vi "Read GPS Data.vi"(0 "VISA resource name":refnum<visa-resource-name>, 5 "Timeout (3000 ms)":u32=3000, 11 "error in (no error)":errorcluster) -> (2 "Speed Over Ground (knots)":dbl, 3 "Bearing (°)":dbl, 4 "VISA resource name out":refnum<visa-resource-name>, 6 "Time Stamp":timestamp, 8 "Latitude (°)":dbl, 10 "Longitude (°)":dbl, 14 "Altitude (m)":dbl, 15 "error out":errorcluster)   [LabVIEW 2011, in "u-blox 5 Series.lvlib"]
doc: "Reads common GPS information from the u-blox device. This VI reads time, longitude, latitude, altitude, speed, and bearing. See u-blox 5 Series Acquire and Chart GPS Data.vi for an example of how it is used."
uses:
  u-blox 5 Series.lvlib
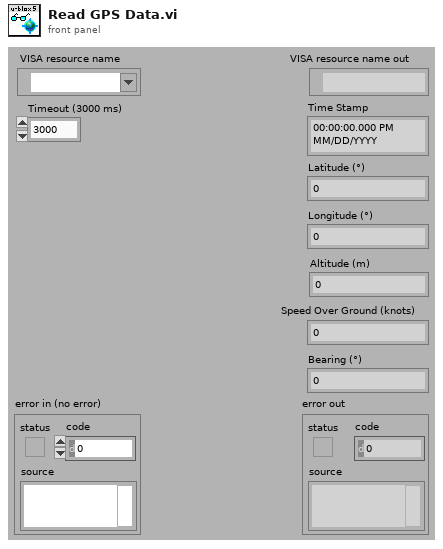
[diagram p1: front panel]
types:
  T1 = cluster{"oldest read timestamp":timestamp, "latitude (deg)":dbl, "longitude (deg)":dbl, "ground speed (knots)":dbl, "true track angle (deg)":dbl, "altitude above mean sea level (m)":dbl}
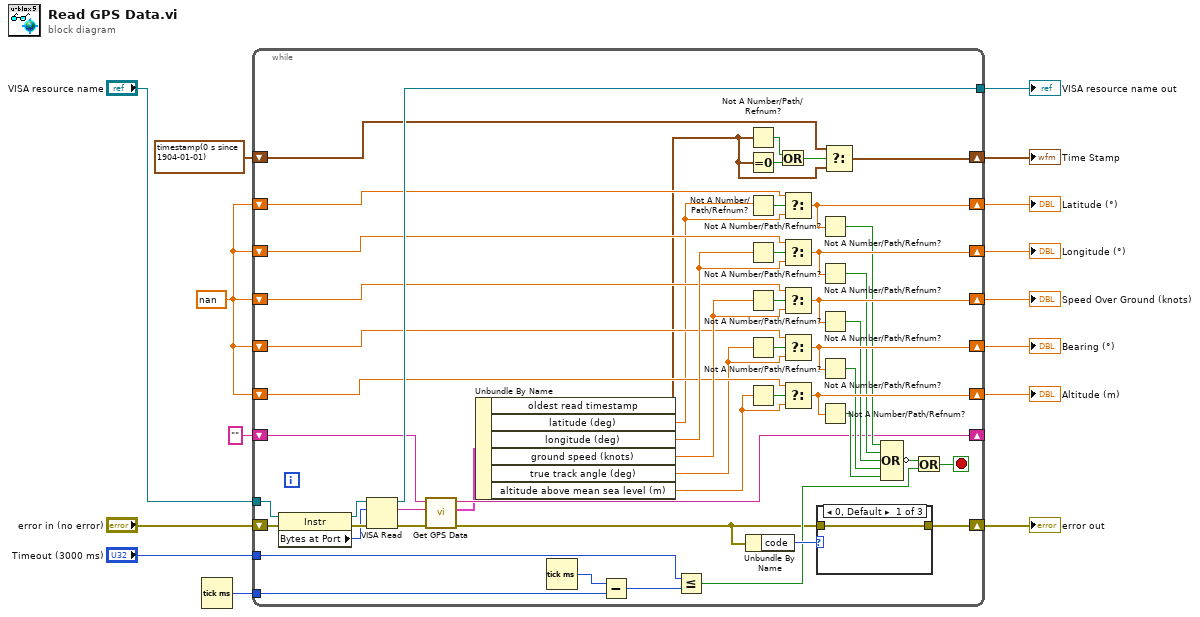
[diagram p0: block diagram]
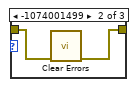
[diagram p2: hidden frame]
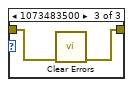
[diagram p3: hidden frame]
diagram:
  w5 = nan
  n1 = Tick Count (ms)() -> (millisecond timer value=w2:u32)
  n2 = while {
    tunnel: "VISA resource name" -> [w26]
    tunnel: [w67] -> w12
    shift-right: [w57] -> w6
    shift-left: timestamp(0 s since 1904-01-01) ("Oldest Read Timestamp") -> [w66]
    shift-right: [w42] -> w11
    shift-left: w5 -> [w65]
    shift-right: [w41] -> w10
    shift-left: w5 -> [w59]
    shift-right: [w21] -> _
    shift-left: "" ("Remaining String after Last Sentence") -> [w20]
    shift-right: [w40] -> w9
    shift-left: w5 -> [w58]
    shift-right: [w39] -> w7
    shift-left: w5 -> [w60]
    shift-right: [w38] -> w8
    shift-left: w5 -> [w61]
    shift-right: [w49] -> w13
    shift-left: "error in (no error)" -> [w25]
    tunnel: w2 -> [w30]
    tunnel: "Timeout (3000 ms)" -> [w22]
    stop <- w43 stop-if-true
    n3 = property class="Instr"(reference=w26, error in=w25) -> (reference out=w27:refnum<visa-resource-name>, error out=w24:errorcluster, "Bytes at Port"=w23:u32)
    n4 = VISA Read(VISA resource name=w27, byte count=w23, error in (no error)=w24) -> (VISA resource name out=w67:refnum<visa-resource-name>, read buffer=w19:string, error out=w18:errorcluster)  [unwired: 1 out]
    n5 = call "Get GPS Data.vi"("error in (no error)"=w18, "sensor data"=w19, "previous partial sentence"=w20) -> ("error out"=w17:errorcluster, "GPS data"=w16:T1, "remaining partial sentence"=w21:string)  [unwired: 6 in]
    n6 = Unbundle By Name(w16) -> ("oldest read timestamp"=w52:timestamp, "latitude (deg)"=w56:dbl, "longitude (deg)"=w64:dbl, "ground speed (knots)"=w63:dbl, "true track angle (deg)"=w51:dbl, "altitude above mean sea level (m)"=w62:dbl)
    n7 = Tick Count (ms)() -> (millisecond timer value=w31:u32)
    n8 = Subtract(x=w31, y=w30) -> (x-y=w29:u32)
    n9 = Less Or Equal?(x=w22, y=w29) -> (x <= y?=w28:bool)
    n10 = Unbundle By Name(w17) -> ("code"=w50:i32)
    n11 = Not A Number/Path/Refnum?(number/path/refnum=w52) -> (NaN/Path/Refnum?=w54:bool)
    n12 = Equal To 0?(x=w52) -> (x = 0?=w53:bool)
    n13 = Not A Number/Path/Refnum?(number/path/refnum=w56) -> (NaN/Path/Refnum?=w48:bool)
    n14 = Not A Number/Path/Refnum?(number/path/refnum=w64) -> (NaN/Path/Refnum?=w47:bool)
    n15 = Not A Number/Path/Refnum?(number/path/refnum=w63) -> (NaN/Path/Refnum?=w44:bool)
    n16 = Not A Number/Path/Refnum?(number/path/refnum=w51) -> (NaN/Path/Refnum?=w45:bool)
    n17 = Not A Number/Path/Refnum?(number/path/refnum=w62) -> (NaN/Path/Refnum?=w46:bool)
    n18 = Or(x=w54, y=w53) -> (x .or. y?=w55:bool)
    n19 = Select(t=w65, s=w48, f=w56) -> (s? t:f=w42:dbl)
    n20 = Select(t=w59, s=w47, f=w64) -> (s? t:f=w41:dbl)
    n21 = Select(t=w58, s=w44, f=w63) -> (s? t:f=w40:dbl)
    n22 = Select(t=w60, s=w45, f=w51) -> (s? t:f=w39:dbl)
    n23 = Select(t=w61, s=w46, f=w62) -> (s? t:f=w38:dbl)
    n24 = case shown="0, Default" w50 {
      tunnel: w17 -> [w68 w70 w72]
      tunnel: [w68 w69 w71] -> w49
      frame 0, Default {
      }
      frame -1074001499 {
        n25 = call <vilib>:"Clear Errors.vi"("error in (no error)"=w70) -> ("error out"=w69:errorcluster)  [unwired: 6 out]
      }
      frame 1073483500 {
        n26 = call <vilib>:"Clear Errors.vi"("error in (no error)"=w72) -> ("error out"=w71:errorcluster)  [unwired: 6 out]
      }
    }
    n27 = Not A Number/Path/Refnum?(number/path/refnum=w42) -> (NaN/Path/Refnum?=w37:bool)
    n28 = Not A Number/Path/Refnum?(number/path/refnum=w41) -> (NaN/Path/Refnum?=w35:bool)
    n29 = Not A Number/Path/Refnum?(number/path/refnum=w40) -> (NaN/Path/Refnum?=w33:bool)
    n30 = Not A Number/Path/Refnum?(number/path/refnum=w39) -> (NaN/Path/Refnum?=w34:bool)
    n31 = Not A Number/Path/Refnum?(number/path/refnum=w38) -> (NaN/Path/Refnum?=w36:bool)
    n32 = Select(t=w66, s=w55, f=w52) -> (s? t:f=w57:timestamp)
    n33 = Compound Arithmetic op=OR(w37, w35, w33, w34, w36) -> (invert w32:bool)
    n34 = Or(x=w32, y=w28) -> (x .or. y?=w43:bool)
  }
  "error out" <- w13
  "VISA resource name out" <- w12
  "Latitude (°)" <- w11
  "Longitude (°)" <- w10
  "Speed Over Ground (knots)" <- w9
  "Bearing (°)" <- w7
  "Altitude (m)" <- w8
  "Time Stamp" <- w6
